vi "BT_Discover.vi"(11 "Device Name":string="ESP32") -> (0 "error out":errorcluster, 1 "device list":T2(array[cluster]), 2 "Device Found?":bool, 3 "Device Address":string, 4 "service list":T1(array[cluster]))   [LabVIEW 2016]
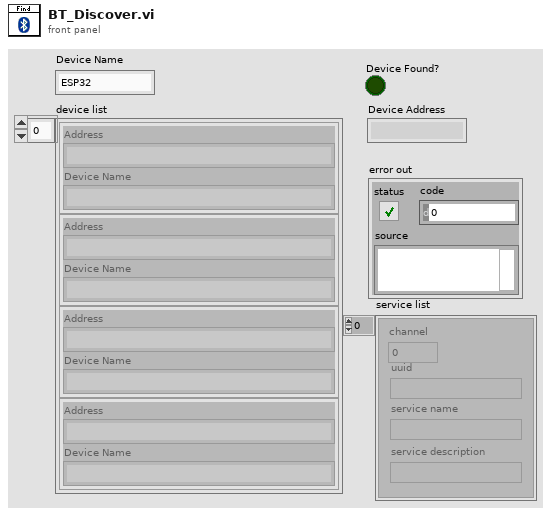
[diagram p1: front panel]
types:
  T1 = cluster{"channel":u16, "uuid":string, "service name":string, "service description":string}[]
  T2 = cluster{"Address":string, "Device Name":string}[]
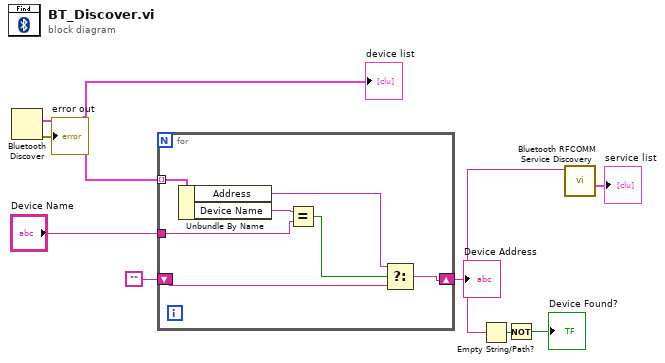
[diagram p0: block diagram]
diagram:
  n1 = Bluetooth Discover() -> (0:→"error out":errorcluster, 2:w7:T2)  [unwired: 2 in, 1 out]
  "device list" <- w7
  n2 = for {
    tunnel: "Device Name" -> [w13]
    tunnel: w7 -> [w15] mode=indexing
    shift-right: [w12] -> w2
    shift-left: "" -> [w11]
    n3 = Unbundle By Name(w15) -> ("Address"=w10:string, "Device Name"=w14:string)
    n4 = Equal?(x=w14, y=w13) -> (x = y?=w9:bool)
    n5 = Select(t=w10, s=w9, f=w11) -> (s? t:f=w12:string)
  }
  "Device Address" <- w2
  n6 = Empty String/Path?(string/path=w2) -> (empty?=w5:bool)
  n7 = Not(x=w5) -> (.not. x?=→"Device Found?":bool)
  n8 = call <vilib>:"Bluetooth RFCOMM Service Discovery.vi"("address in"=w2) -> ("service list"=→"service list":T1)  [unwired: 3 in, 3 out]
